vi "wait_test_01.vi"() -> ()   [LabVIEW 2011]
uses:
  wait_globals.vi
panel:
  out "Total Wait Time (m:s)":string
  out "Waiting":bool
  out "Wait Time Remaining(m:s)":string
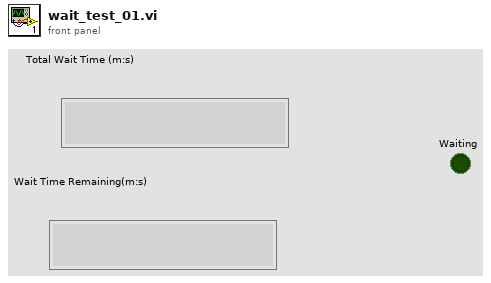
[diagram p1: front panel]
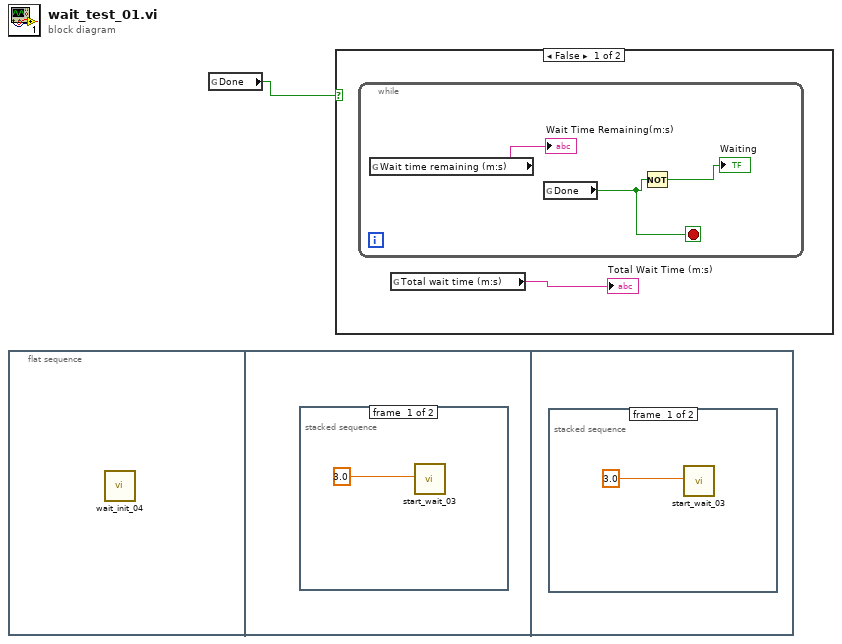
[diagram p0: block diagram]
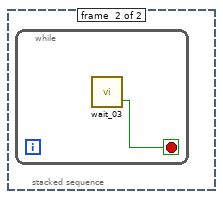
[diagram p3: hidden frame]
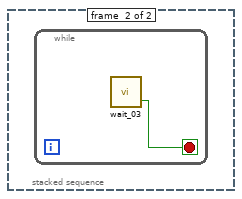
[diagram p4: hidden frame]
diagram:
  n1 = flat-sequence {
    frame #0 {
      n2 = call "wait_init_04.vi"() -> ()  [unwired: 1 in]
    }
    frame #1 {
      n3 = stacked-sequence {
        frame #0 {
          n4 = call "start_wait_03.vi"("Total wait time (s)"=3.0 ("Wait (s)")) -> ()
        }
        frame #1 {
          n5 = while {
            stop <- w3 stop-if-true
            n6 = call "wait_03.vi"() -> ("Done"=w3:bool)  [unwired: 1 in, 1 out]
          }
        }
      }
    }
    frame #2 {
      n7 = stacked-sequence {
        frame #0 {
          n8 = call "start_wait_03.vi"("Total wait time (s)"=3.0 ("Wait (s)")) -> ()
        }
        frame #1 {
          n9 = while {
            stop <- w5 stop-if-true
            n10 = call "wait_03.vi"() -> ("Done"=w5:bool)  [unwired: 1 in, 1 out]
          }
        }
      }
    }
  }
  n11 = global read "wait_globals.vi" "Done"() -> (w1:bool)
  n12 = case shown="False" w1 {
    frame False {
      n13 = global read "wait_globals.vi" "Total wait time (m:s)"() -> (→"Total Wait Time (m:s)":string)
    }
    frame True {
    }
  }
  n14 = while {
    stop <- w7 stop-if-true
    n15 = global read "wait_globals.vi" "Wait time remaining (m:s)"() -> (→"Wait Time Remaining(m:s)":string)
    n16 = global read "wait_globals.vi" "Done"() -> (w7:bool)
    n17 = Not(x=w7) -> (.not. x?=→"Waiting":bool)
  }
